vi "DAQprime.vi"(2 "error in":errorcluster, 3 "DAQ Card/Channels":i32[](array[numeric])=[3, 8], 4 "Tree DVR In":refnum<data-value>) -> (0 "error out":errorcluster)   [LabVIEW 2014]
uses:
  <vilib>/MDSplus/Classes/Tree_Class/Tree.lvclass
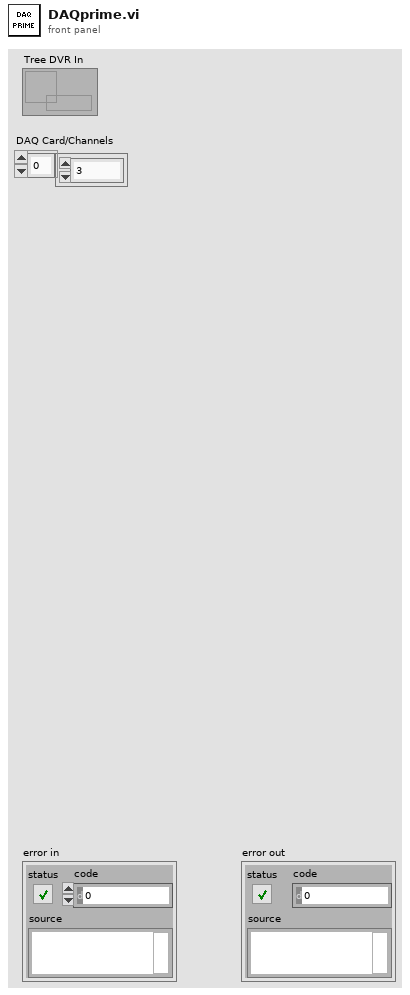
[diagram p1: front panel]
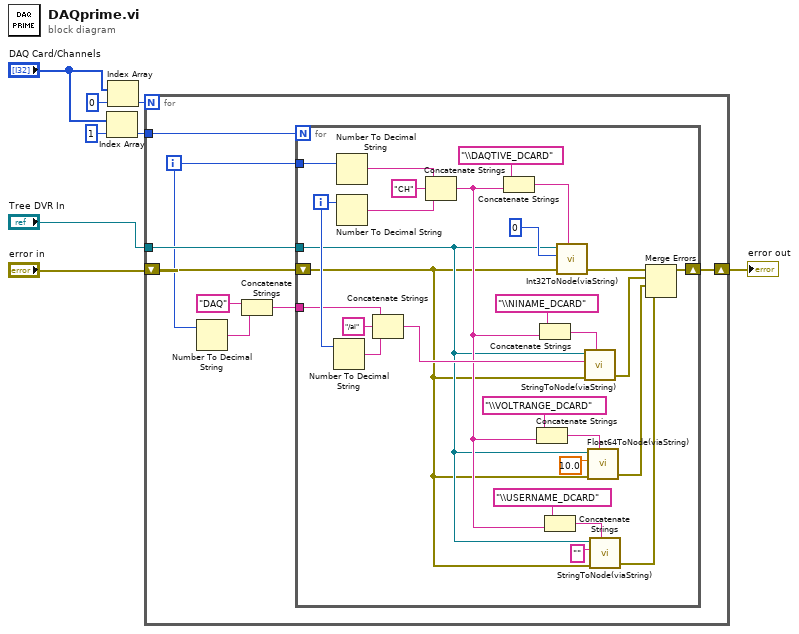
[diagram p0: block diagram]
diagram:
  n1 = Index Array(array="DAQ Card/Channels", index=1) -> (element=w2:i32)
  n2 = Index Array(array="DAQ Card/Channels", index=0) -> (element=w3:i32)
  n3 = for {
    N: w3 -> [_]
    shift-right: [w15] -> w6
    shift-left: "error in" -> [w16]
    tunnel: "Tree DVR In" -> [w14]
    tunnel: w2 -> [w13]
    i -> [w10]
    n4 = Number To Decimal String(number=w10) -> (decimal integer string=w12:string)  [unwired: 1 in]
    n5 = Concatenate Strings("DAQ", w12) -> (w9:string)
    n6 = for {
      N: w13 -> [_]
      tunnel: w10 -> [w42]
      shift-right: [w35] -> w15
      shift-left: w16 -> [w19]
      tunnel: w14 -> [w20]
      tunnel: w9 -> [w29]
      i -> [w30]
      n7 = Number To Decimal String(number=w30) -> (decimal integer string=w31:string)  [unwired: 1 in]
      n8 = Number To Decimal String(number=w42) -> (decimal integer string=w43:string)  [unwired: 1 in]
      n9 = Number To Decimal String(number=w30) -> (decimal integer string=w41:string)  [unwired: 1 in]
      n10 = Concatenate Strings(w29, "/ai" ("string"), w31) -> (w28:string)
      n11 = Concatenate Strings(w43, "CH" ("string"), w41) -> (w21:string)
      n12 = Concatenate Strings("\\DAQTIVE_DCARD" ("string"), w21) -> (w38:string)
      n13 = Concatenate Strings("\\VOLTRANGE_DCARD" ("string"), w21) -> (w27:string)
      n14 = Concatenate Strings("\\NINAME_DCARD" ("string"), w21) -> (w37:string)
      n15 = Concatenate Strings("\\USERNAME_DCARD" ("string"), w21) -> (w23:string)
      n16 = call "Int32ToNode(viaString).vi"("Tree DVR in"=w20, "I32 in"=0, "error in (no error)"=w19, "NodePath"=w38) -> ("error out"=w33:errorcluster)  [unwired: 1 in, 2 out]
      n17 = call "StringToNode(viaString).vi"("Tree DVR in"=w20, "String value in"=w28, "error in (no error)"=w19, "NodePath"=w37) -> ("error out"=w34:errorcluster)  [unwired: 2 in, 1 out]
      n18 = call "Float64ToNode(viaString).vi"("Tree DVR in"=w20, "DBL in"=10.0, "error in"=w19, "NodePath"=w27) -> ("error out"=w24:errorcluster)  [unwired: 2 in, 1 out]
      n19 = call "StringToNode(viaString).vi"("Tree DVR in"=w20, "String value in"="", "error in (no error)"=w19, "NodePath"=w23) -> ("error out"=w18:errorcluster)  [unwired: 2 in, 1 out]
      n20 = Merge Errors(w33, w34, w24, w18) -> (w35:errorcluster)
    }
  }
  "error out" <- w6
